vi "Test Galil Terminal.vi"() -> ()   [LabVIEW 2011]
panel:
  in  "Delay Time (s)":dbl=1.0
  out "Error Query Connection":errorcluster
  out "Error Galil Command":errorcluster
  out "Error Initialize Galil":errorcluster
  in  "stop":bool
  out "Output String 3":string
  out "timeout_ms":i32=500
  out "address":string="192.168.1.10"
  in  "Galil.IGalil":refnum<k7>
  in  "Initial Encoder Counts":string
  in  "Command Input":string
  out "Command Output":string
  in  "Close Command Input":string
  out "Close Command Output":string
  out "Error Close Galil":errorcluster
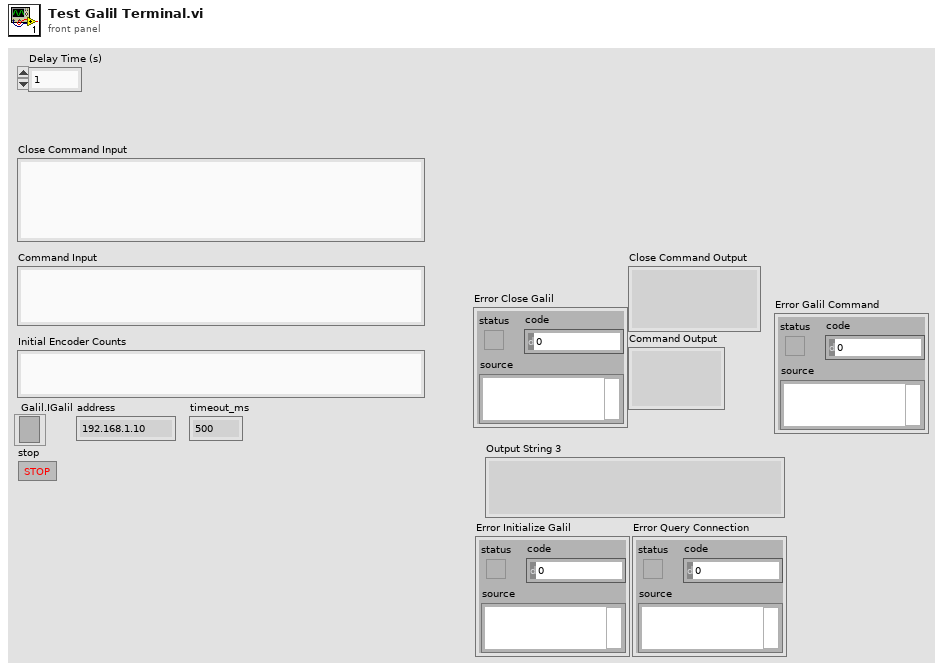
[diagram p1: front panel]
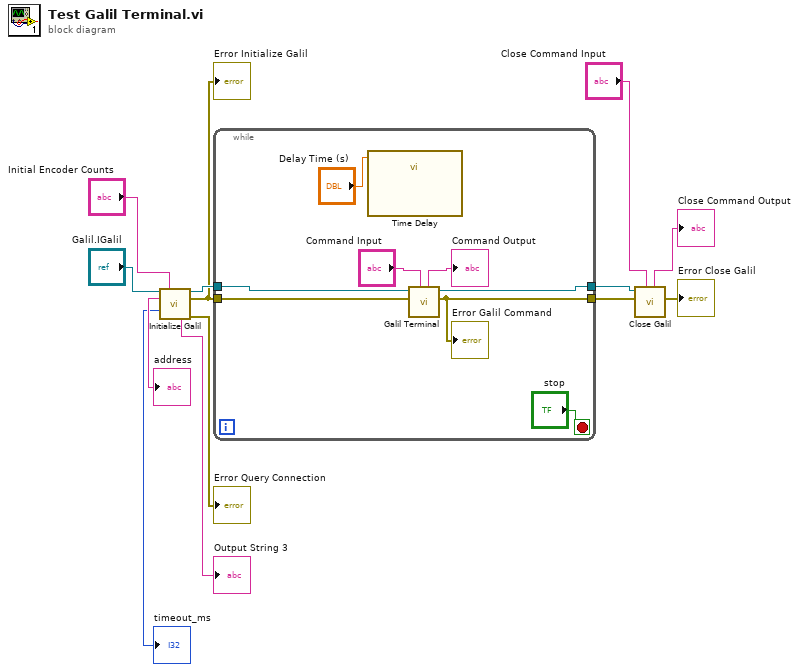
[diagram p0: block diagram]
diagram:
  n1 = call "Initialize Galil.vi"("Galil.IGalil"="Galil.IGalil", "Initial Encoder Counts"="Initial Encoder Counts") -> ("reference out 3"=w13:refnum<k7>, "address"=→"address":string, "error out 3"=w12:errorcluster, "timeout_ms"=→"timeout_ms":i32, "Output String"=→"Output String 3":string, "Error Query Connection"=→"Error Query Connection":errorcluster)  [unwired: 8 in]
  "Error Initialize Galil" <- w12
  n2 = while {
    tunnel: w13 -> [w21]
    tunnel: w12 -> [w20]
    tunnel: [w19] -> w11
    tunnel: [w18] -> w10
    stop <- "stop" stop-if-true
    n3 = call "Time Delay"("Delay Time (s)"="Delay Time (s)") -> ()  [unwired: 10 in, 1 out]
    n4 = call "Galil Terminal.vi"("Command Input"="Command Input", "Galil Error In"=w20, "reference out 2"=w21) -> ("Galil Error Out"=w18:errorcluster, "reference out 3"=w19:refnum<k7>, "Command Output"=→"Command Output":string)  [unwired: 6 in]
    "Error Galil Command" <- w18
  }
  n5 = call "Close Galil.vi"("Command Input"="Close Command Input", "error out 2"=w10, "reference out 2"=w11) -> ("error out"=→"Error Close Galil":errorcluster, "Output String"=→"Close Command Output":string)  [unwired: 7 in]
